vi "Pre Launch Init.vi"(11 "Jiaxin_Stepper_Controller in":refnum<class "Jiaxin_Stepper_Controller.lvclass">) -> (0 "error out":errorcluster, 3 "Jiaxin_Stepper_Controller out":refnum<class "Jiaxin_Stepper_Controller.lvclass">)   [LabVIEW 2023, in "Jiaxin_Stepper_Controller.lvlib" / "Jiaxin_Stepper_Controller.lvclass"]
doc: "(<B>Filename</B>: Actor Framework.lvlib:Actor.lvclass:Pre Launch Init.vi)\n\nDefines behavior that occurs after the Launch Nested Actor method is invoked but before the actor's Actor Core method begins running.\n\nBy default, this method does nothing. A descendant class may override it to define behavior."
uses:
  Jiaxin_Stepper_Controller.lvclass
  Jiaxin_Stepper_Controller.lvclass/Jiaxin_Stepper_Controller.ctl
  <vilib>/ActorFramework/Actor/Actor.lvclass
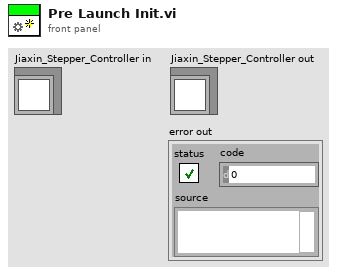
[diagram p1: front panel]
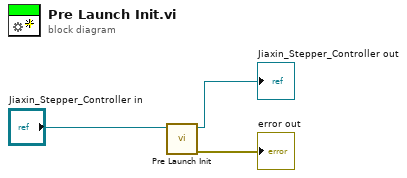
[diagram p0: block diagram]
diagram:
  n1 = call-parent "Pre Launch Init.vi"("Actor in"="Jiaxin_Stepper_Controller in") -> ("error out"=→"error out":errorcluster, "Actor out"=→"Jiaxin_Stepper_Controller out":refnum<class "Jiaxin_Stepper_Controller.lvclass">)  [unwired: 9 in]
